vi "Main.vi"() -> ()   [LabVIEW 2017]
uses:
  <vilib>/DAQmx/read.llb/DAQmx Read (Analog DBL 1Chan 1Samp).vi
  <vilib>/DAQmx/create/channels.llb/DAQmx Create Channel (AI-Voltage-Basic).vi
  <vilib>/DAQmx/create/channels.llb/DAQmx Create Channel (CI-Count Edges).vi
panel:
  in  "Encoder Index":tag="Dev3/port0/line1"
  in  "Encoder B":tag="Dev3/port0/line1"
  in  "Encoder A":tag="Dev3/port0/line1"
  in  "Sonar":tag="Dev3/port0/line1"
  in  "Optical Switch":tag="Dev3/port0/line1"
  in  "Strain":tag="Dev3/port0/line1"
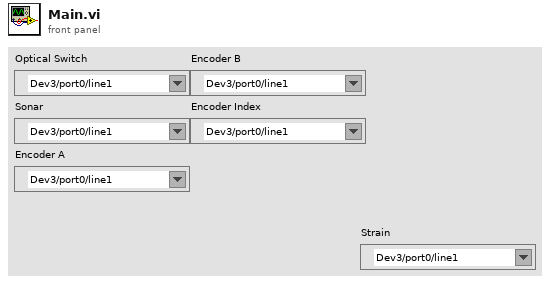
[diagram p1: front panel]
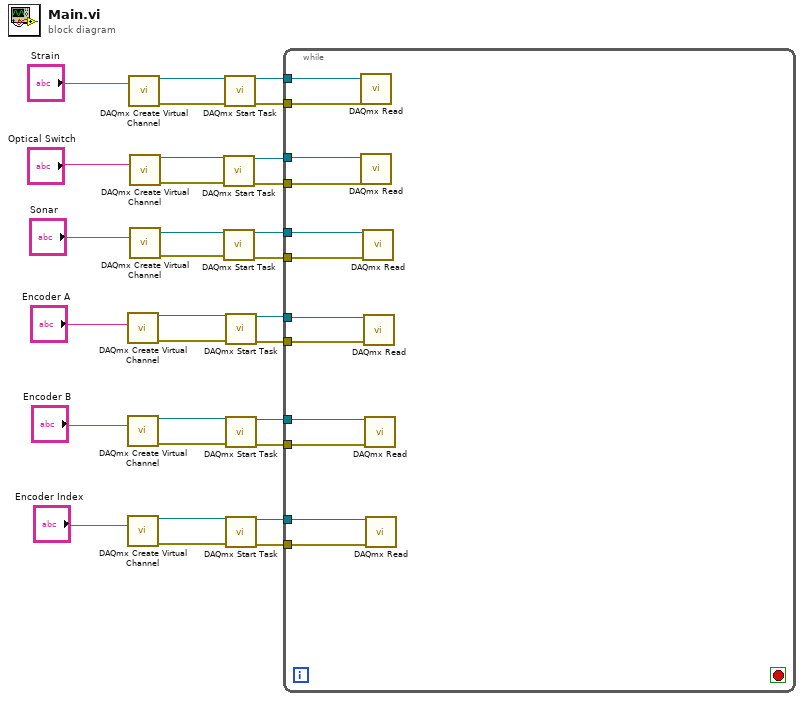
[diagram p0: block diagram]
diagram:
  n1 = call-poly <vilib>:"DAQmx Create Virtual Channel.vi"("counter"="Encoder A") -> ("task out"=w22:refnum<k21>, "error out"=w13:errorcluster)  [unwired: 13 in]
  n2 = call-poly <vilib>:"DAQmx Create Virtual Channel.vi"("counter"="Encoder B") -> ("task out"=w11:refnum<k21>, "error out"=w10:errorcluster)  [unwired: 13 in]
  n3 = call-poly <vilib>:"DAQmx Create Virtual Channel.vi"("counter"="Encoder Index") -> ("task out"=w9:refnum<k21>, "error out"=w8:errorcluster)  [unwired: 13 in]
  n4 = call-poly <vilib>:"DAQmx Create Virtual Channel.vi"("physical channels"="Strain") -> ("task out"=w25:refnum<k21>, "error out"=w17:errorcluster)  [unwired: 13 in]
  n5 = call-poly <vilib>:"DAQmx Create Virtual Channel.vi"("physical channels"="Optical Switch") -> ("task out"=w24:refnum<k21>, "error out"=w18:errorcluster)  [unwired: 13 in]
  n6 = call-poly <vilib>:"DAQmx Create Virtual Channel.vi"("physical channels"="Sonar") -> ("task out"=w23:refnum<k21>, "error out"=w15:errorcluster)  [unwired: 13 in]
  n7 = call <vilib>:"DAQmx Start Task.vi"("task/channels in"=w24, "error in"=w18) -> ("task out"=w28:refnum<k21>, "error out"=w16:errorcluster)  [unwired: 12 in]
  n8 = call <vilib>:"DAQmx Start Task.vi"("task/channels in"=w23, "error in"=w15) -> ("task out"=w27:refnum<k21>, "error out"=w14:errorcluster)  [unwired: 12 in]
  n9 = call <vilib>:"DAQmx Start Task.vi"("task/channels in"=w25, "error in"=w17) -> ("task out"=w30:refnum<k21>, "error out"=w29:errorcluster)  [unwired: 12 in]
  n10 = call <vilib>:"DAQmx Start Task.vi"("task/channels in"=w22, "error in"=w13) -> ("task out"=w26:refnum<k21>, "error out"=w12:errorcluster)  [unwired: 12 in]
  n11 = call <vilib>:"DAQmx Start Task.vi"("task/channels in"=w11, "error in"=w10) -> ("task out"=w6:refnum<k21>, "error out"=w5:errorcluster)  [unwired: 12 in]
  n12 = call <vilib>:"DAQmx Start Task.vi"("task/channels in"=w9, "error in"=w8) -> ("task out"=w4:refnum<k21>, "error out"=w3:errorcluster)  [unwired: 12 in]
  n13 = while {
    tunnel: w30 -> [w42]
    tunnel: w29 -> [w41]
    tunnel: w28 -> [w40]
    tunnel: w27 -> [w39]
    tunnel: w26 -> [w38]
    tunnel: w16 -> [w37]
    tunnel: w14 -> [w36]
    tunnel: w12 -> [w35]
    tunnel: w6 -> [w34]
    tunnel: w5 -> [w33]
    tunnel: w4 -> [w32]
    tunnel: w3 -> [w31]
    stop <- _ stop-if-true
    n14 = call-poly <vilib>:"DAQmx Read.vi"("task/channels in"=w42, "error in"=w41) -> ()  [unwired: 11 in, 3 out]
    n15 = call-poly <vilib>:"DAQmx Read.vi"("task/channels in"=w40, "error in"=w37) -> ()  [unwired: 11 in, 3 out]
    n16 = call-poly <vilib>:"DAQmx Read.vi"("task/channels in"=w39, "error in"=w36) -> ()  [unwired: 11 in, 3 out]
    n17 = call-poly <vilib>:"DAQmx Read.vi"("task/channels in"=w38, "error in"=w35) -> ()  [unwired: 11 in, 3 out]
    n18 = call-poly <vilib>:"DAQmx Read.vi"("task/channels in"=w34, "error in"=w33) -> ()  [unwired: 11 in, 3 out]
    n19 = call-poly <vilib>:"DAQmx Read.vi"("task/channels in"=w32, "error in"=w31) -> ()  [unwired: 11 in, 3 out]
  }
